vi "MGI Row[] to Details.vi"(10 "Selected Row[]":i32[](array[numeric]), 11 "MGI Error Reporter Dialog In":refnum<class "MGI Error Reporter Dialog.lvclass">) -> (1 "Call Chain[occurred..TopLevel]":string[](array[string]), 2 "Error Details":string, 3 "MGI Error Reporter Dialog Out":refnum<class "MGI Error Reporter Dialog.lvclass">)   [LabVIEW 2016, in "MGI Error Reporter Dialog.lvclass"]
doc: "Converts the specified error to a call chain and a details string which includes possible error causes.\n\nAuthored by Shawn Walpole\nsupport@mooregoodideas.com\nwww.mooregoodideas.com\n\nCopyright (c) 2013, Moore Good Ideas, Inc.\n\nAll rights reserved.\n\nRedistribution and use in source and binary forms, with or without modification, are permitted provided that the following conditions are met:\n\n * Redistributions of source code must retain the above copyright notice, this list of conditions and the following disclaimer.\n * Redistributions in binary form must reproduce the above copyright notice, this list of conditions and the following disclaimer in the documentation and/or other materials provided with the distribution.\n * Neither the name of Moore Good Ideas, Inc. nor the names of its contributors may be used to endorse or promote products derived from this software without specific prior written permission.\n\nTHIS SOFTWARE IS PROVIDED BY THE COPYRIGHT HOLDERS AND CONTRIBUTORS \"AS IS\" AND ANY EXPRESS OR IMPLIED WARRANTIES, INCLUDING, BUT NOT LIMITED TO, THE IMPLIED WARRANTIES OF MERCHANTABILITY AND FITNESS FOR A PARTICULAR PURPOSE ARE DISCLAIMED. IN NO EVENT SHALL THE COPYRIGHT OWNER OR CONTRIBUTORS BE LIABLE FOR ANY DIRECT, INDIRECT, INCIDENTAL, SPECIAL, EXEMPLARY, OR CONSEQUENTIAL DAMAGES (INCLUDING, BUT NOT LIMITED TO, PROCUREMENT OF SUBSTITUTE GOODS OR SERVICES; LOSS OF USE, DATA, OR PROFITS; OR BUSINESS INTERRUPTION) HOWEVER CAUSED AND ON ANY THEORY OF LIABILITY, WHETHER IN CONTRACT, STRICT LIABILITY, OR TORT (INCLUDING NEGLIGENCE OR OTHERWISE) ARISING IN ANY WAY OUT OF THE USE OF THIS SOFTWARE, EVEN IF ADVISED OF THE POSSIBILITY OF SUCH DAMAGE."
uses:
  <userlib>/_MGI/Error Reporter/MGI Error Reporter Dialog/MGI Error Reporter Dialog.lvclass
  C:/Program Files (x86)/National Instruments/LabVIEW 2016/user.lib/_MGI/Error Reporter/MGI Error Reporter Base/MGI Error Reporter Base.lvclass
  <userlib>/_MGI/Error Reporter/MGI Error Reporter Dialog/MGI Error Reporter Dialog.lvclass/MGI Error Reporter Dialog.ctl
  <userlib>/_MGI/Error Reporter/MGI Error Reporter Dialog/MGI ERD LB Row Base/MGI ERD LB Row Base.lvclass
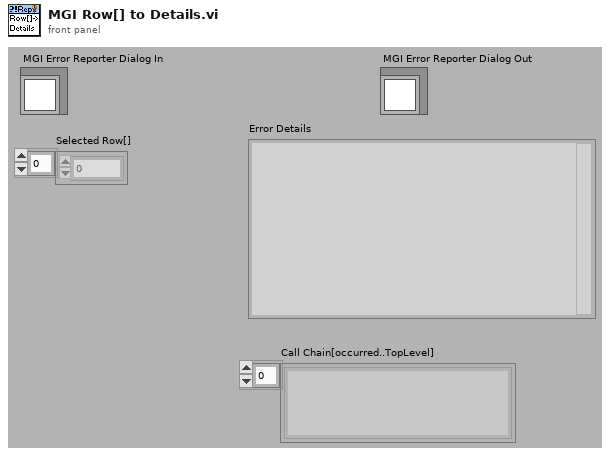
[diagram p1: front panel]
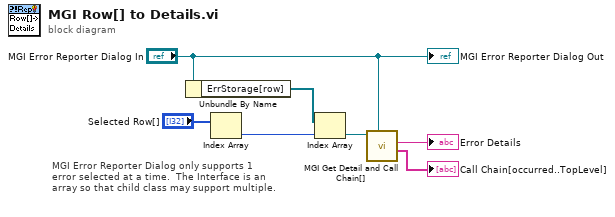
[diagram p0: block diagram]
diagram:
  # "MGI Error Reporter Dialog only supports 1 error selected at a time.  The Interface is an array so that child class may support multiple."
  n1 = Unbundle By Name("MGI Error Reporter Dialog In") -> ("ErrStorage[row]"=w6:refnum<class "MGI ERD LB Row Base.lvclass">[])
  n2 = Index Array(array="Selected Row[]") -> (element=w5:i32)  [unwired: 1 in]
  n3 = Index Array(array=w6, index=w5) -> (element=w4:refnum<class "MGI ERD LB Row Base.lvclass">)
  n4 = call-dynamic "MGI Get Detail and Call Chain[].vi"("MGI Error Reporter Base In"="MGI Error Reporter Dialog In", "MGI ERD LB Row Base in"=w4) -> ("Call Chain[..Top Level]"=→"Call Chain[occurred..TopLevel]":string[], "Details"=→"Error Details":string)  [unwired: 1 in, 7 out]
  "MGI Error Reporter Dialog Out" <- "MGI Error Reporter Dialog In"
